vi "Compute Protocol Matches a Special Scheme.vi"(11 "Constructor String Parser In":T1) -> (0 "error IO":errorcluster, 2 "Special Scheme":bool, 3 "Constructor String Parser":T1)   [LabVIEW 2020, in "Stream.lvlib" / "URLPattern.lvclass"]
uses:
  URLPattern.lvclass
  Constructor String Parser.ctl
  Token.ctl
  Token Type.ctl
  URL Pattern Init.ctl
  Parser State.ctl
  Canonicalize Protocol.vi
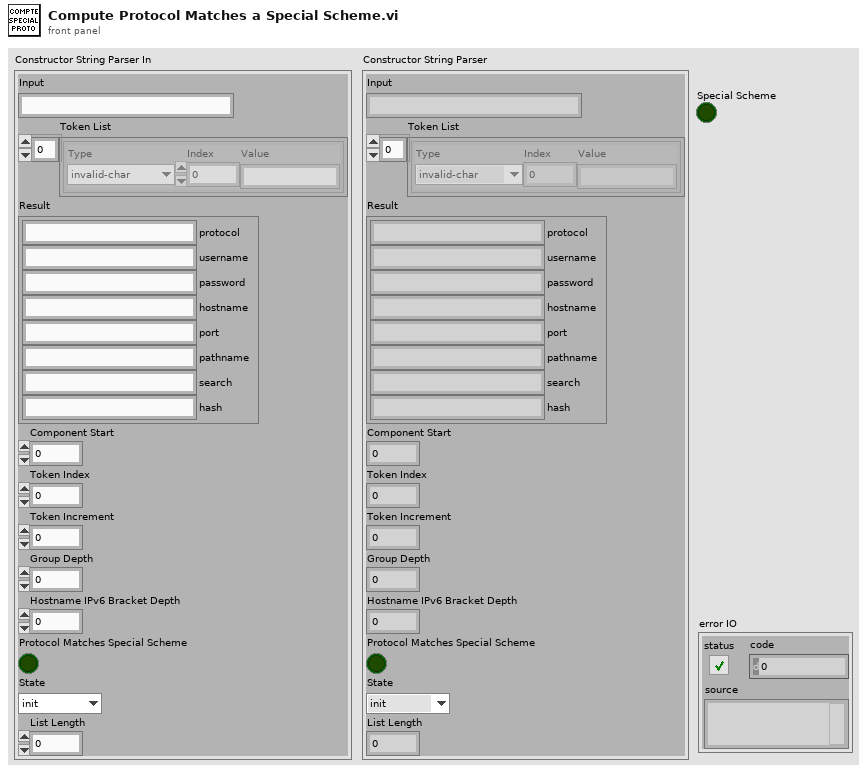
[diagram p1: front panel]
types:
  T1 = typedef "Stream.lvlib/URLPattern.lvclass/Constructor String Parser.ctl" = cluster{"Input":string, "Token List":T2[], "Result":T4, "Component Start":i32, "Token Index":i32, "Token Increment":i32, "Group Depth":i32, "Hostname IPv6 Bracket Depth":i32, "Protocol Matches Special Scheme":bool, "State":T5, "List Length":i32}
  T2 = typedef "Stream.lvlib/URLPattern.lvclass/Token.ctl" = cluster{"Type":T3, "Index":i32, "Value":string}
  T3 = typedef "Stream.lvlib/URLPattern.lvclass/Token Type.ctl" = enum16{"invalid-char", "open", "close", "regexp", "name", "char", "escaped-char", "other-modifier", "asterisk", "end"}
  T4 = typedef "Stream.lvlib/URLPattern.lvclass/URL Pattern Init.ctl" = cluster{"protocol":string, "username":string, "password":string, "hostname":string, "port":string, "pathname":string, "search":string, "hash":string}
  T5 = typedef "Stream.lvlib/URLPattern.lvclass/Parser State.ctl" = enum16{"init", "protocol", "authority", "username", "password", "hostname", "port", "pathname", "search", "hash", "done"}
  T6 = typedef "Stream.lvlib/URLPattern.lvclass/Component.ctl" = cluster{"Pattern String":string, "Regular Expression":string, "Name List":string[]}
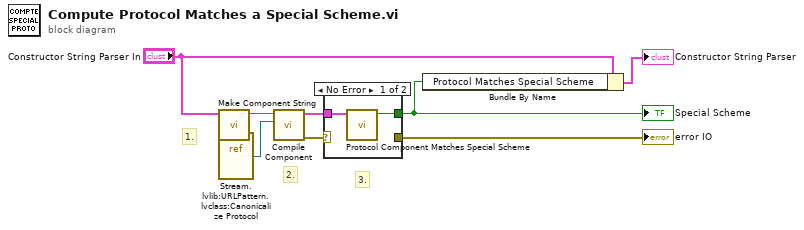
[diagram p0: block diagram]
diagram:
  # "3."
  # "2."
  # "1."
  n1 = call "Make Component String.vi"("Constructor String Parser"="Constructor String Parser In") -> ("Component String"=w8:string)  [unwired: 9 in, 1 out]
  n2 = vi-ref "Stream.lvlib:URLPattern.lvclass:Canonicalize Protocol.vi"() -> (w7:refnum<vi>)
  n3 = call "Compile Component.vi"("Encoding Callback"=w7, "Input"=w8) -> ("error IO"=w5:errorcluster, "Component"=w6:T6)  [unwired: 8 in]
  n4 = case shown="No Error" w5 {
    selector: w5 -> [_ w11]
    tunnel: w6 -> [w10 _]
    tunnel: [_ w11] -> w4
    tunnel: [w9 _] -> w2
    frame No Error {
      n5 = call "Protocol Component Matches Special Scheme.vi"("Component"=w10) -> ("Special Scheme"=w9:bool)  [unwired: 10 in]
    }
    frame Error {
    }
  }
  "error IO" <- w4
  "Special Scheme" <- w2
  n6 = Bundle By Name(cluster="Constructor String Parser In", "Protocol Matches Special Scheme"=w2) -> (→"Constructor String Parser":T1)
